vi "FindEyes_DEPRECATED.vi"(8 "error in (no error)":errorcluster, 10 "image":picture, 11 "reference in":refnum<class "ImageFacialDetection.lvclass">) -> (0 "error out":errorcluster, 2 "image with Eyes":picture, 3 "reference out":refnum<class "ImageFacialDetection.lvclass">)   [LabVIEW 2017]
doc: "uses the image classification in python with openCV to detect faces in an image using Haar Cascades"
uses:
  ImageFacialDetection.lvclass
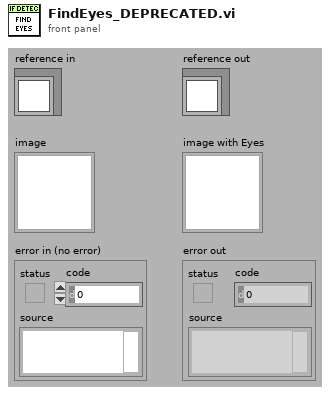
[diagram p1: front panel]
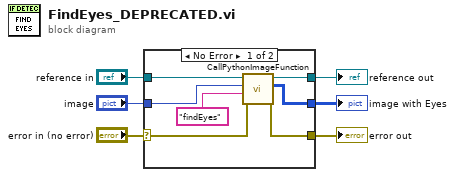
[diagram p0: block diagram]
diagram:
  n1 = case shown="No Error" "error in (no error)" {
    selector: "error in (no error)" -> [w8 w15]
    tunnel: [w7 w15] -> w5
    tunnel: [w12 w14] -> w3
    tunnel: "reference in" -> [w13 w14]
    tunnel: "image" -> [w11 _]
    tunnel: [w9 _] -> w1
    frame No Error {
      n2 = call "CallPythonImageFunction.vi"("error in (no error)"=w8, "Function or Method Name"="findEyes", "Python Image Data in"=w11, "reference in"=w13) -> ("error out"=w7:errorcluster, "Python Image Data out"=w9:u8[][][], "reference out"=w12:refnum<class "ImageFacialDetection.lvclass">)  [unwired: 5 in]
    }
    frame Error {
    }
  }
  "error out" <- w5
  "reference out" <- w3
  "image with Eyes" <- w1
